vi "BRig_Host_v0,52__noGlobal.vi"() -> ()   [LabVIEW 2014]
uses:
  <vilib>/WebDAVClient/Advanced/SessionHandle.ctl
  BRig_Host__global__stopHost.vi
  <vilib>/Utility/file.llb/Write To Spreadsheet File (DBL).vi
  <vilib>/WebDAVClient/NI_WebDAV.lvlib
panel:
  out "writeError":bool
  out "error IO":errorcluster
  out "error_loopP_loadSettings":errorcluster caption="error out"
  out "testCmdList":u16[][](array[numeric])
  in  "ClosedLoop":bool
  in  "module":string=" module1 "
  in  "input_updateTrial_subsequent":u16
  in  "input_updateTrial_first":u16
  in  "input_forceUpdate":bool
  in  "ClosedLoop":u16[](array[numeric])
  in  "testNewLaserSettings":bool
  in  "LoadSettings":bool
  in  "DisplayNumber":u16
  out "XY Graph":cluster{u16[], u16[]}[](graph)
  in  "threshold_2":u16=600
  in  "threshold_1":u16=300
  in  "Port (F=A/B, T=C)":bool
  out "I_ExpRun":bool
  out "TCP_connection":bool
  in  "stopHost":bool
  # "Port Switch\nToggle TRUE if debugging"
  # "# Trials Displayed\n( 0 = all )"
  # "Selection\nTime Thresholds"
  # "Exp Run\nIn Progress"
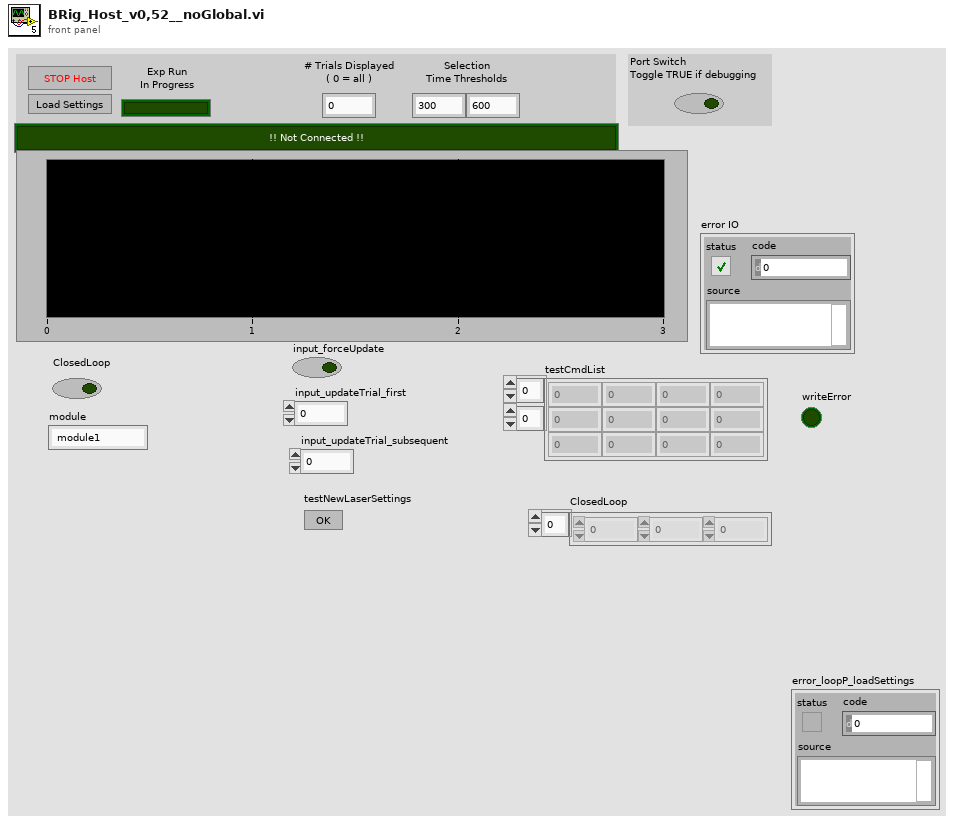
[diagram p1: front panel]
types:
  T1 = typedef "NI_WebDAV.lvlib/SessionHandle.ctl" = refnum<k1>
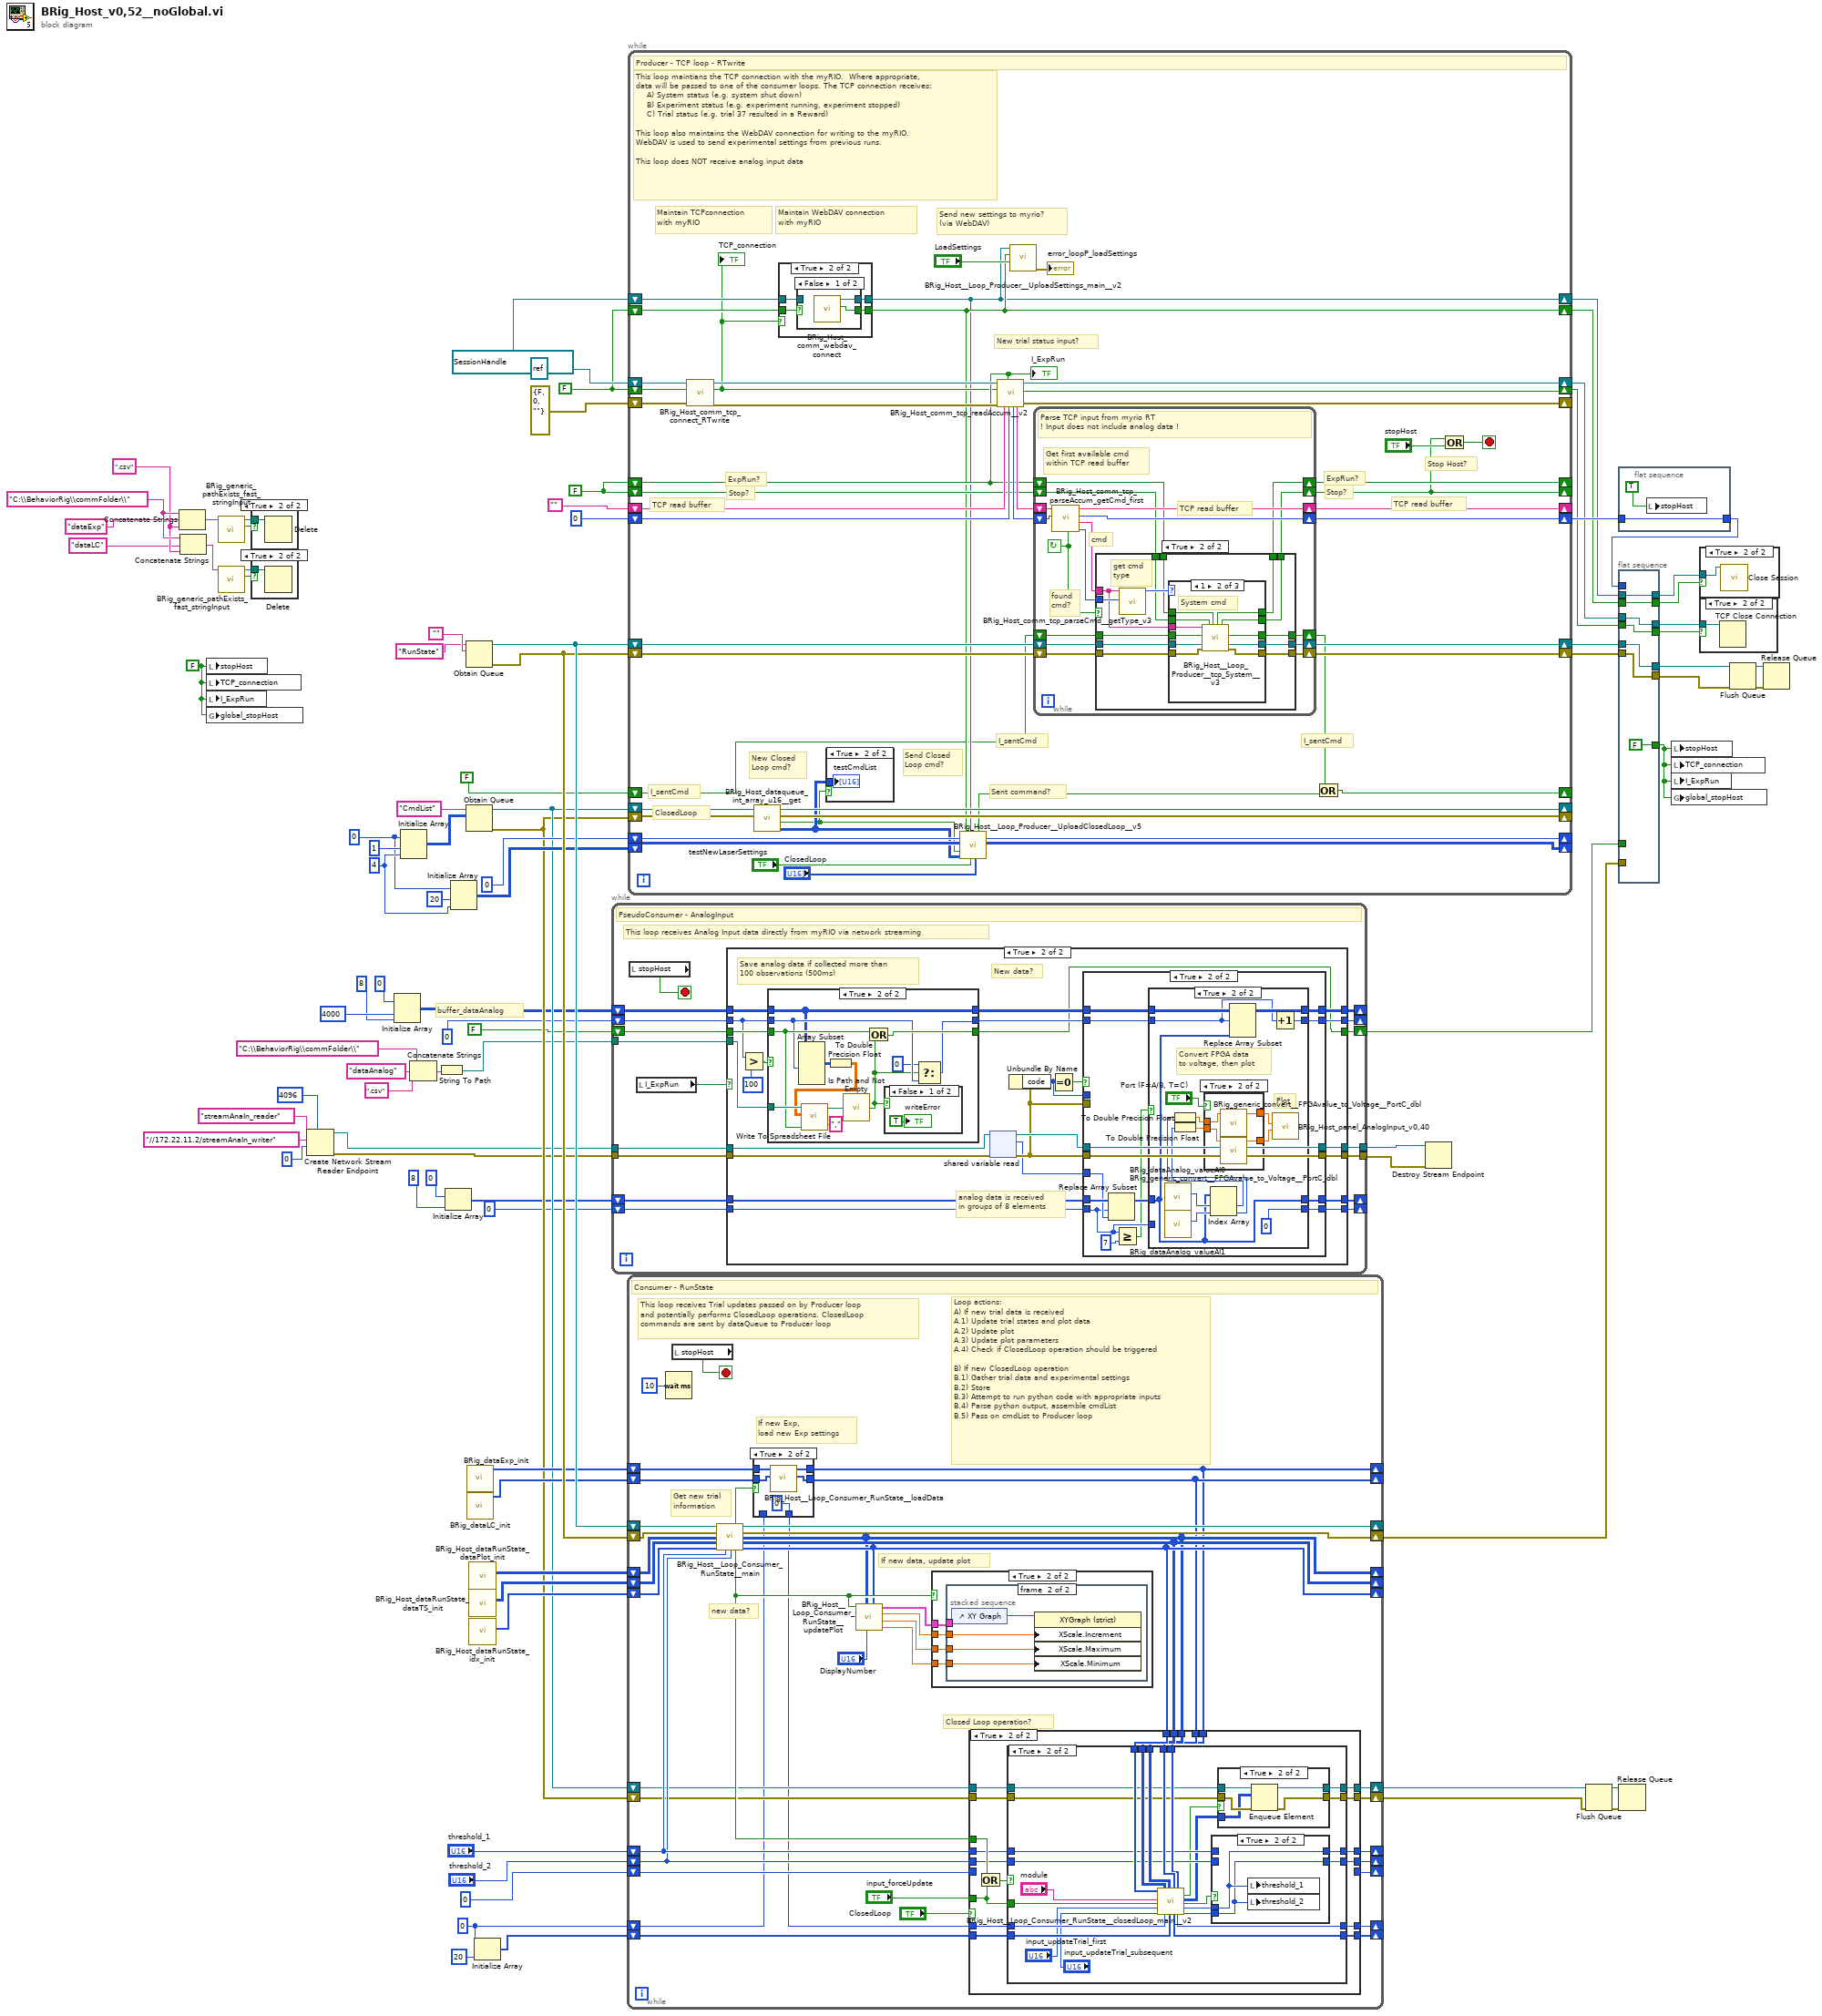
[diagram p0: block diagram]
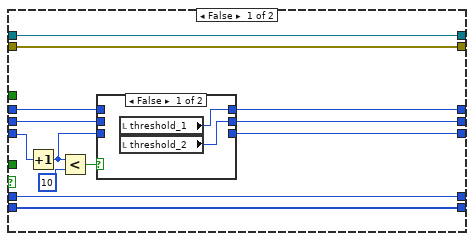
[diagram p6: hidden frame]
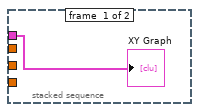
[diagram p13: hidden frame]
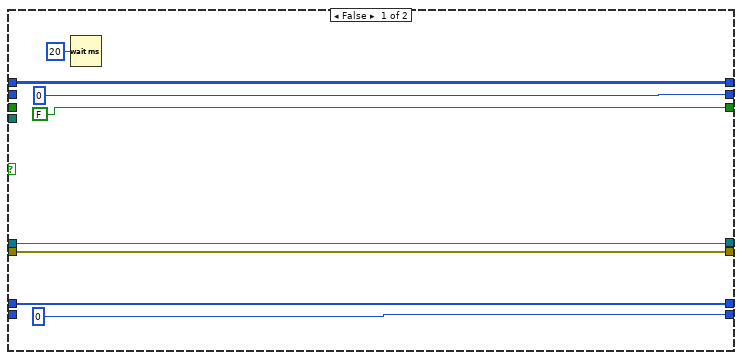
[diagram p14: hidden frame]
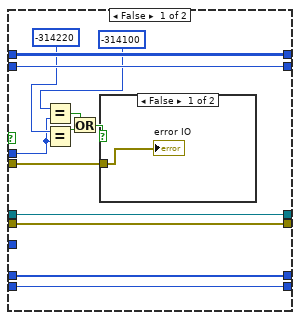
[diagram p15: hidden frame]
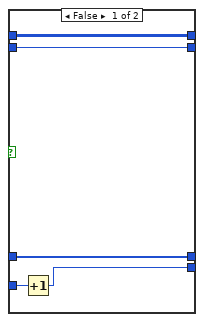
[diagram p17: hidden frame]
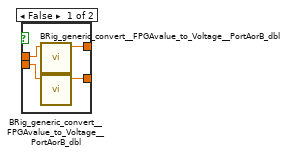
[diagram p18: hidden frame]
diagram:
  w25 = u16 0 ("element")
  w26 = 4 ("dimension size")
  w42 = u16 0
  w54 = ".csv" ("string")
  w55 = "C:\\BehaviorRig\\commFolder\\"
  w67 = T1 refnum items=["Session NI_WebDAV"] ("session handle")
  w85 = FALSE ("stopHost")
  w86 = FALSE
  w68 = FALSE
  # "buffer_dataAnalog"
  n1 = Concatenate Strings(w55, "dataExp" ("string"), w54) -> (w49:string)
  n2 = Concatenate Strings(w55, "dataLC" ("string"), w54) -> (w46:string)
  n3 = local write "stopHost"(w85) -> ()
  n4 = local write "TCP_connection"(w85) -> ()
  n5 = local write "I_ExpRun"(w85) -> ()
  n6 = global write "BRig_Host__global__stopHost.vi" "global_stopHost"(w85) -> ()
  n7 = call "BRig_generic_pathExists_fast_stringInput.vi"("input_filePath"=w49) -> ("output_Iexist"=w51:bool, "output_filePath"=w50:path)  [unwired: 8 in, 1 out]
  n8 = call "BRig_generic_pathExists_fast_stringInput.vi"("input_filePath"=w46) -> ("output_Iexist"=w47:bool, "output_filePath"=w48:path)  [unwired: 8 in, 1 out]
  n9 = case shown="True" w51 {
    tunnel: w50 -> [_ w91]
    frame False {
    }
    frame True {
      n10 = Delete(path (use dialog)=w91) -> ()  [unwired: 4 in, 3 out]
    }
  }
  n11 = case shown="True" w47 {
    tunnel: w48 -> [_ w92]
    frame False {
    }
    frame True {
      n12 = Delete(path (use dialog)=w92) -> ()  [unwired: 4 in, 3 out]
    }
  }
  n13 = Create Network Stream Reader Endpoint(7:4096 ("reader buffer size"), 9:u16 0 ("element"), 10:"//172.22.11.2/streamAnaIn_writer" ("writer url"), 11:"streamAnaIn_reader" ("reader name")) -> (0:w9:errorcluster, 3:w10:refnum<k21>)  [unwired: 3 in]
  n14 = Initialize Array(u16 0 ("element"), 4000 ("dimension size"), 8 ("dimension size")) -> (w21:u16[][])
  n15 = Initialize Array(w25, 1 ("dimension size"), w26) -> (w37:u16[][])
  n16 = Concatenate Strings("C:\\BehaviorRig\\commFolder\\" ("string"), "dataAnalog" ("input_filename"), ".csv" ("string")) -> (w18:string)
  n17 = String To Path(string=w18) -> (path=w15:path)
  n18 = Initialize Array(u16 0 ("element"), 8 ("dimension size")) -> (w2:u16[])
  n19 = Initialize Array(w25, 20 ("dimension size"), w26) -> (w56:u16[][])
  n20 = Obtain Queue(name (unnamed)="RunState", element data type="") -> (queue out=w77:refnum<queue>, error out=w76:errorcluster)  [unwired: 3 in, 1 out]
  n21 = Obtain Queue(name (unnamed)="CmdList", element data type=w37) -> (queue out=w36:refnum<queue>, error out=w35:errorcluster)  [unwired: 3 in, 1 out]
  n22 = call "BRig_dataExp_init.vi"() -> ("output_dataExp"=w45:u16[])  [unwired: 11 in]
  n23 = call "BRig_dataLC_init.vi"() -> ("output_dataLC"=w44:u16[])  [unwired: 11 in]
  n24 = call "BRig_Host_dataRunState_dataPlot_init.vi"() -> ("output_dataPlot"=w73:u16[][])  [unwired: 11 in]
  n25 = call "BRig_Host_dataRunState_dataTS_init.vi"() -> ("output_dataTS"=w72:u16[][])  [unwired: 11 in]
  n26 = call "BRig_Host_dataRunState_idx_init.vi"() -> ("output_idx"=w71:i32[])  [unwired: 11 in]
  n27 = Initialize Array(w42, 20 ("dimension size")) -> (w40:u16[])
  n28 = while {
    shift-right: [w107] -> _
    shift-left: w21 -> [w109]
    shift-right: [w106] -> _
    shift-left: 0 -> [w108]
    tunnel: w15 -> [w105]
    shift-right: [w103] -> w13
    shift-left: FALSE -> [w104]
    tunnel: w10 -> [w101]
    tunnel: w9 -> [w100]
    tunnel: [w99] -> w7
    tunnel: [w98] -> w6
    shift-right: [w95] -> _
    shift-left: w2 -> [w97]
    shift-right: [w94] -> _
    shift-left: 0 ("element") -> [w96]
    stop <- w93 stop-if-true
    # "This loop receives Analog Input data directly from myRIO via network streaming"
    # "PseudoConsumer - AnalogInput"
    n29 = local read "stopHost"() -> (w93:bool)
    n30 = local read "I_ExpRun"() -> (w102:bool)
    n31 = case shown="True" w102 {
      tunnel: w109 -> [w116 w140]
      tunnel: w108 -> [_ w126]
      tunnel: [w116 w135] -> w107
      tunnel: [0 w133] -> w106
      tunnel: w105 -> [_ w138]
      tunnel: w104 -> [_ w139]
      tunnel: [FALSE w123] -> w103
      tunnel: w101 -> [w113 w132]
      tunnel: w100 -> [w112 w131]
      tunnel: [w113 w129] -> w99
      tunnel: [w112 w127] -> w98
      tunnel: w97 -> [w111 w121]
      tunnel: w96 -> [_ w120]
      tunnel: [w111 w119] -> w95
      tunnel: [0 ("element") w118] -> w94
      frame False {
        n32 = Wait (ms)(milliseconds to wait=u32 20) -> ()  [unwired: 1 out]
      }
      frame True {
        # "analog data is received\nin groups of 8 elements"
        # "New data?"
        # "Save analog data if collected more than\n100 observations (500ms)"
        n33 = Greater?(x=w126, y=100) -> (0:w141:bool)
        n34 = case shown="True" w141 {
          tunnel: w140 -> [w200 w203]
          tunnel: [w200 w203] -> w136
          tunnel: w126 -> [w199 w205]
          tunnel: w139 -> [w198 w207]
          tunnel: [w199 w204] -> w134
          tunnel: [w198 w206] -> w123
          tunnel: w138 -> [_ w212]
          frame False {
          }
          frame True {
            n35 = Array Subset(array=w203, length (row)=w205) -> (w211:u16[][])  [unwired: 3 in]
            n36 = To Double Precision Float(number=w211) -> (double precision float=w210:dbl[][])
            n37 = call-poly <vilib>:"Write To Spreadsheet File.vi"("delimiter (\\t)"="," ("delimiter (\\t)"), "append to file? (new file:F)"=w207, "2D data"=w210, "file path (dialog if empty)"=w212) -> ("new file path (Not A Path if cancelled)"=w208:path)  [unwired: 4 in]
            n38 = call <vilib>:"Is Path and Not Empty.vi"("path"=w208) -> ("Is Path and Not Empty?"=w201:bool)  [unwired: 4 in]
            n39 = Or(x=w207, y=w201) -> (x .or. y?=w206:bool)
            n40 = case shown="False" w201 {
              frame False {
                "writeError" <- TRUE ("writeError")
              }
              frame True {
              }
            }
            n41 = Select(t=0, s=w201, f=w205) -> (s? t:f=w204:i32)
          }
        }
        n42 = shared-variable-read(w132, w131) -> (w130:refnum<k21>, w128:errorcluster, w122:u16)  [unwired: 1 in, 1 out]
        n43 = Unbundle By Name(w128) -> ("code"=w124:i32)
        n44 = Equal To 0?(x=w124) -> (x = 0?=w137:bool)
        n45 = case shown="True" w137 {
          tunnel: w136 -> [w154 w169]
          tunnel: [w154 w168] -> w135
          tunnel: w134 -> [w153 w167]
          tunnel: [w153 w166] -> w133
          tunnel: w128 -> [w151 _]
          tunnel: w130 -> [w150 w165]
          tunnel: [w150 w165] -> w129
          tunnel: w128 -> [w149 w164]
          tunnel: [w149 w164] -> w127
          tunnel: w124 -> [w148 _]
          tunnel: w122 -> [_ w162]
          tunnel: w121 -> [w143 w163]
          tunnel: w120 -> [w142 w160]
          tunnel: [w143 w157] -> w119
          tunnel: [w142 w159] -> w118
          frame False {
            n46 = Equal?(x=-314100, y=w148) -> (x = y?=w146:bool)
            n47 = Equal?(x=-314220, y=w148) -> (x = y?=w145:bool)
            n48 = Or(x=w146, y=w145) -> (x .or. y?=w144:bool)
            n49 = case shown="False" w144 {
              tunnel: w151 -> [w155 _]
              frame False {
                "error IO" <- w155
              }
              frame True {
              }
            }
          }
          frame True {
            n50 = Replace Array Subset(array=w163, new element=w162, index=w160) -> (w158:u16[])
            n51 = Greater Or Equal?(x=w160, y=7) -> (x >= y?=w156:bool)
            n52 = case shown="True" w156 {
              tunnel: w169 -> [w174 w189]
              tunnel: [w174 w188] -> w168
              tunnel: w167 -> [w173 w187]
              tunnel: [w173 w186] -> w166
              tunnel: w160 -> [w172 _]
              tunnel: [w171 0 ("y")] -> w159
              tunnel: w158 -> [w170 w177]
              tunnel: [w170 w177] -> w157
              frame False {
                n53 = Increment(x=w172) -> (x+1=w171:i32)
              }
              frame True {
                # "Convert FPGA data\nto voltage, then plot"
                # "Plot"
                n54 = call "BRig_dataAnalog_valueAI0.vi"() -> ("output_valueAI0"=w179:i32)  [unwired: 11 in]
                n55 = call "BRig_dataAnalog_valueAI1.vi"() -> ("output_valueAI1"=w180:i32)  [unwired: 11 in]
                n56 = Index Array(array=w177, index #1=w179, index #2=w180) -> (element #1=w176:u16, element #2=w175:u16)
                n57 = To Double Precision Float(number=w176) -> (double precision float=w181:dbl)
                n58 = To Double Precision Float(number=w175) -> (double precision float=w182:dbl)
                n59 = case shown="True" "Port (F=A/B, T=C)" {
                  tunnel: w181 -> [w191 w197]
                  tunnel: w182 -> [w190 w196]
                  tunnel: [w193 w195] -> w184
                  tunnel: [w192 w194] -> w183
                  frame False {
                    n60 = call "BRig_generic_convert__FPGAvalue_to_Voltage__PortAorB_dbl.vi"("input_FPGAvalue_PortAorB"=w191) -> ("output_voltage"=w193:dbl)  [unwired: 10 in]
                    n61 = call "BRig_generic_convert__FPGAvalue_to_Voltage__PortAorB_dbl.vi"("input_FPGAvalue_PortAorB"=w190) -> ("output_voltage"=w192:dbl)  [unwired: 10 in]
                  }
                  frame True {
                    n62 = call "BRig_generic_convert__FPGAvalue_to_Voltage__PortC_dbl.vi"("input_FPGAvalue_PortC"=w197) -> ("output_voltage"=w195:dbl)  [unwired: 10 in]
                    n63 = call "BRig_generic_convert__FPGAvalue_to_Voltage__PortC_dbl.vi"("input_FPGAvalue_PortC"=w196) -> ("output_voltage"=w194:dbl)  [unwired: 10 in]
                  }
                }
                n64 = Replace Array Subset(array=w189, new element=w177, index (row)=w187) -> (w188:u16[][])  [unwired: 1 in]
                n65 = Increment(x=w187) -> (x+1=w186:i32)
                n66 = call "BRig_Host_panel_AnalogInput_v0,40.vi"("graph_ai1"=w183, "graph_ai0"=w184) -> ()  [unwired: 10 in]
              }
            }
          }
        }
      }
    }
  }
  n67 = while {
    shift-right: [w246] -> _
    shift-left: w77 -> [w247]
    shift-right: [w244] -> w30
    shift-left: w76 -> [w245]
    shift-right: [w227] -> _
    shift-left: w73 -> [w243]
    shift-right: [w228] -> _
    shift-left: w72 -> [w242]
    shift-right: [w229] -> _
    shift-left: w71 -> [w241]
    shift-right: [w237] -> _
    shift-left: "threshold_1" -> [w236]
    shift-right: [w235] -> _
    shift-left: "threshold_2" -> [w234]
    shift-right: [w225] -> _
    shift-left: w45 -> [w239]
    shift-right: [w226] -> _
    shift-left: w44 -> [w238]
    shift-right: [w219] -> _
    shift-left: w42 -> [w217]
    shift-right: [w231] -> _
    shift-left: u8 0 -> [w232]
    shift-right: [w218] -> _
    shift-left: w40 -> [w215]
    shift-right: [w222] -> w32
    shift-left: w36 -> [w224]
    shift-right: [w221] -> w31
    shift-left: w35 -> [w223]
    stop <- w214 stop-if-true
    # "Closed Loop operation?"
    # "Loop actions:\nA) If new trial data is received\nA.1) Update trial states and plot data\nA.2) Update plot\nA.3) Update plot parameters\nA.4) Check if ClosedLoop operation should be triggered\n\nB) If new ClosedLoop operation\nB.1) Gather trial data and experimental settings\nB.2) Store\nB.3) Attempt to run python code with appropriate inputs\nB.4) Parse python output, assemble cmdList\nB.5) Pass on cmdList to Producer loop"
    # "This loop receives Trial updates passed on by Producer loop\nand potentially performs ClosedLoop operations. ClosedLoop\ncommands are sent by dataQueue to Producer loop"
    # "If new data, update plot"
    # "If new Exp,\nload new Exp settings"
    # "new data?"
    # "Get new trial\ninformation"
    # "Consumer - RunState"
    n68 = Wait (ms)(milliseconds to wait=u32 10) -> ()  [unwired: 1 out]
    n69 = local read "stopHost"() -> (w214:bool)
    n70 = call "BRig_Host__Loop_Consumer_RunState__main.vi"("input_hDataQueue"=w247, "input_errorDataQueue"=w245, "input_dataPlot"=w243, "input_dataTS"=w242, "input_idx"=w241, "threshold_1"=w236, "threshold_2"=w234) -> ("output_ExpStart"=w240:bool, "output_hDataQueue"=w246:refnum<queue>, "output_errorDataQueue"=w244:errorcluster, "output_dataPlot"=w227:u16[][], "output_dataTS"=w228:u16[][], "output_updatePlot"=w230:bool, "output_idx"=w229:i32[])  [unwired: 2 in]
    n71 = case shown="True" w240 {
      tunnel: w239 -> [w337 w339]
      tunnel: [w337 w342] -> w225
      tunnel: w238 -> [w336 w340]
      tunnel: [w336 w341] -> w226
      tunnel: w217 -> [w335 _]
      tunnel: [w335 u16 0] -> w216
      frame False {
      }
      frame True {
        n72 = call "BRig_Host__Loop_Consumer_RunState__loadData.vi"("input_dataLC"=w340, "input_dataExp"=w339) -> ("output_dataLC"=w341:u16[], "output_dataExp"=w342:u16[])  [unwired: 8 in]
      }
    }
    n73 = call "BRig_Host__Loop_Consumer_RunState__updatePlot.vi"("input_idx"=w229, "input_DisplayNumber"="DisplayNumber", "input_dataPlot"=w227, "input_updatePlot"=w230) -> ("output_X_min"=w250:dbl, "output_X_max"=w249:dbl, "output_X_inc"=w248:dbl, "XY Graph"=w251:cluster{u16[], u16[]}[])  [unwired: 4 in]
    n74 = case shown="True" w230 {
      tunnel: w251 -> [_ w346]
      tunnel: w250 -> [_ w345]
      tunnel: w249 -> [_ w344]
      tunnel: w248 -> [_ w343]
      frame False {
      }
      frame True {
        n75 = stacked-sequence {
          tunnel: w346 -> [w347 _]
          tunnel: w345 -> [_ w350]
          tunnel: w344 -> [_ w349]
          tunnel: w343 -> [_ w348]
          frame #0 {
            "XY Graph" <- w347
          }
          frame #1 {
            n76 = control-ref of="XY Graph"() -> (w351:refnum<vi>)
            n77 = property class="XYGraph (strict)"(reference=w351, "XScale.Increment"=w348, "XScale.Maximum"=w349, "XScale.Minimum"=w350) -> ()  [unwired: 1 in, 2 out]
          }
        }
      }
    }
    n78 = case shown="True" "ClosedLoop" {
      tunnel: [w261 w284] -> w237
      tunnel: w236 -> [w262 w285]
      tunnel: [w260 w282] -> w235
      tunnel: w234 -> [w263 w283]
      tunnel: w232 -> [w266 _]
      tunnel: [w259 _] -> w231
      tunnel: w216 -> [w257 w289]
      tunnel: [w257 w287] -> w219
      tunnel: w215 -> [w256 w288]
      tunnel: [w256 w286] -> w218
      tunnel: w230 -> [_ w291]
      tunnel: w229 -> [_ w281]
      tunnel: w228 -> [_ w280]
      tunnel: w227 -> [_ w279]
      tunnel: w226 -> [_ w278]
      tunnel: w225 -> [_ w277]
      tunnel: w224 -> [w255 w276]
      tunnel: w223 -> [w254 w275]
      tunnel: [w255 w274] -> w222
      tunnel: [w254 w273] -> w221
      tunnel: "input_forceUpdate" -> [_ w272]
      frame False {
        n79 = Increment(x=w266) -> (x+1=w258:u8)
        n80 = Less?(x=w258, y=u8 10) -> (x < y?=w264:bool)
        n81 = case shown="False" w264 {
          tunnel: w263 -> [_ w270]
          tunnel: w262 -> [_ w271]
          tunnel: [w268 w271] -> w261
          tunnel: [w267 w270] -> w260
          tunnel: [_ w269] -> w259
          tunnel: w258 -> [_ w269]
          frame False {
            n82 = local read "threshold_1"() -> (w268:u16)
            n83 = local read "threshold_2"() -> (w267:u16)
          }
          frame True {
          }
        }
      }
      frame True {
        n84 = Or(x=w291, y=w272) -> (x .or. y?=w290:bool)
        n85 = case shown="True" w290 {
          tunnel: w272 -> [_ w320]
          tunnel: w289 -> [w297 w323]
          tunnel: w288 -> [w296 w322]
          tunnel: [w297 w316] -> w287
          tunnel: [w296 w317] -> w286
          tunnel: w285 -> [w295 w310]
          tunnel: [w295 w306] -> w284
          tunnel: w283 -> [w294 w309]
          tunnel: [w294 w305] -> w282
          tunnel: w281 -> [_ w315]
          tunnel: w280 -> [_ w314]
          tunnel: w279 -> [_ w313]
          tunnel: w278 -> [_ w312]
          tunnel: w277 -> [_ w311]
          tunnel: w276 -> [w293 w303]
          tunnel: w275 -> [w292 w301]
          tunnel: [w293 w302] -> w274
          tunnel: [w292 w300] -> w273
          frame False {
          }
          frame True {
            n86 = call "BRig_Host__Loop_Consumer_RunState__closedLoop_main__v2.vi"("input_idx"=w315, "input_module"="module", "input_forceUpdate"=w320, "input_updateTrial_first"="input_updateTrial_first", "input_updateTrial_subsequent"="input_updateTrial_subsequent", "input_dataTS"=w314, "input_updateID"=w323, "input_dataPlot"=w313, "input_trialList"=w322, "input_dataLC"=w312, "input_dataExp"=w311) -> ("output_trialList"=w317:u16[], "output_updateID"=w316:u16, 15:"output_cmdList"=w298:bool, 16:"output_cmdList"=w299:u16[][], "output_thres"=w304:bool, "output_thres1"=w308:u16, "output_thres2"=w307:u16)  [unwired: 2 in]
            n87 = case shown="True" w304 {
              tunnel: w310 -> [w332 _]
              tunnel: w309 -> [w331 _]
              tunnel: w308 -> [_ w334]
              tunnel: w307 -> [_ w333]
              tunnel: [w332 w334] -> w306
              tunnel: [w331 w333] -> w305
              frame False {
              }
              frame True {
                n88 = local write "threshold_1"(w334) -> ()
                n89 = local write "threshold_2"(w333) -> ()
              }
            }
            n90 = case shown="True" w298 {
              tunnel: w303 -> [w325 w330]
              tunnel: [w325 w327] -> w302
              tunnel: w301 -> [w324 w329]
              tunnel: [w324 w326] -> w300
              tunnel: w299 -> [_ w328]
              frame False {
              }
              frame True {
                n91 = Enqueue Element(queue=w330, element=w328, error in (no error)=w329) -> (queue out=w327:refnum<queue>, error out=w326:errorcluster)  [unwired: 1 in, 1 out]
              }
            }
          }
        }
      }
    }
  }
  n92 = while {
    shift-right: [w378] -> w61
    shift-left: w68 -> [w398]
    shift-right: [w393] -> w62
    shift-left: refnum<k5> refnum ("output_hTCP") -> [w397]
    shift-right: [w392] -> _
    shift-left: errorcluster {"status"=FALSE, "code"=0, "source"=""} ("output_error") -> [w396]
    shift-right: [w387] -> _
    shift-left: "" ("input_strAccum") -> [w391]
    shift-right: [w386] -> w75
    shift-left: 0 ("input_count") -> [w390]
    shift-right: [w385] -> _
    shift-left: w86 -> [w363]
    shift-right: [w361] -> _
    shift-left: w86 -> [w383]
    shift-right: [w380] -> w81
    shift-left: w77 -> [w382]
    shift-right: [w379] -> w80
    shift-left: w76 -> [w381]
    shift-right: [w358] -> w66
    shift-left: w68 -> [w377]
    shift-right: [w357] -> w65
    shift-left: w67 -> [w376]
    shift-right: [w368] -> _
    shift-left: w56 -> [w369]
    shift-right: [w352] -> _
    shift-left: 0 -> [w370]
    shift-right: [w372] -> _
    shift-left: w36 -> [w374]
    shift-right: [w371] -> _
    shift-left: w35 -> [w373]
    shift-right: [w353] -> _
    shift-left: FALSE -> [w356]
    stop <- w360 stop-if-true
    # "ClosedLoop"
    # "TCP read buffer"
    # "TCP read buffer"
    # "I_sentCmd"
    # "Sent command?"
    # "I_sentCmd"
    # "I_sentCmd"
    # "Stop Host?"
    # "Send Closed\nLoop cmd?"
    # "New Closed\nLoop cmd?"
    # "New trial status input?"
    # "ExpRun?"
    # "Stop?"
    # "This loop maintians the TCP connection with the myRIO.  Where appropriate,\ndata will be passed to one of the consumer loops. The TCP connection receives:\n    A) System status (e.g. system shut down)\n    B) Experiment status (e.g. experiment running, experiment stopped)\n    C) Trial status (e.g. trial 37 resulted in a Reward)\n\nThis loop also maintains the WebDAV connection for writing to the myRIO.\nWebDAV is used to send experimental settings from previous runs.\n\nThis loop does NOT receive analog input data"
    # "Send new settings to myrio?\n(via WebDAV)"
    # "ExpRun?"
    # "Stop?"
    # "Maintain TCPconnection\nwith myRIO"
    # "Maintain WebDAV connection\nwith myRIO"
    # "Producer - TCP loop - RTwrite"
    n93 = call "BRig_Host_comm_tcp_connect_RTwrite.vi"("input_error"=w396, "input_connected"=w398, "input_hTCP"=w397) -> ("output_error"=w394:errorcluster, "output_connected"=w362:bool, "output_hTCP"=w395:refnum<k5>)  [unwired: 5 in, 1 out]
    "TCP_connection" <- w362
    n94 = call "BRig_Host_dataqueue_int_array_u16__get.vi"("input_erroDataQueue"=w373, "input_hDataQueue"=w374) -> (0:"output_data"=w365:u16[][], 1:"output_data"=w364:bool, "output_errorDataQueue"=w371:errorcluster, "output_hDataQueue"=w372:refnum<queue>)  [unwired: 6 in]
    n95 = case shown="True" w362 {
      tunnel: w377 -> [w403 w411]
      tunnel: [w402 w410] -> w358
      tunnel: w376 -> [w401 w409]
      tunnel: [w400 w408] -> w357
      frame False {
        n96 = case shown="True" w403 {
          selector: w403 -> [w405 _]
          tunnel: [w405 FALSE] -> w402
          tunnel: w401 -> [w404 w406]
          tunnel: [w404 _] -> w400
          frame False {
          }
          frame True {
            n97 = call <vilib>:"Close Session.vi"("session handle"=w406) -> ()  [unwired: 14 in, 1 out]
          }
        }
      }
      frame True {
        n98 = case shown="False" w411 {
          selector: w411 -> [_ w415]
          tunnel: [w412 w415] -> w410
          tunnel: w409 -> [_ w414]
          tunnel: [w413 w414] -> w408
          frame False {
            n99 = call "BRig_Host_comm_webdav_connect.vi"() -> ("output_Iconnected"=w412:bool, "output_hSession"=w413:T1)  [unwired: 9 in, 1 out]
          }
          frame True {
          }
        }
      }
    }
    n100 = case shown="True" w364 {
      tunnel: w365 -> [_ w399]
      frame False {
      }
      frame True {
        "testCmdList" <- w399
      }
    }
    n101 = call "BRig_Host__Loop_Producer__UploadClosedLoop__v5.vi"("input_arrayBuffer_length"=w370, "input_arrayBuffer"=w369, 4:"input_cmdList"=w364, 5:"input_cmdList"=w365, "input_webdav_status"=w358, "session handle"=w357, "testNewLaserSettings"="testNewLaserSettings", "input_array_LaserSettings"="ClosedLoop") -> ("Sent"=w354:bool, "output_arrayBuffer_length"=w352:i32, "output_arrayBuffer"=w368:u16[][])  [unwired: 9 in]
    n102 = call "BRig_Host_comm_tcp_readAccum__v2.vi"("input_handle_TCP"=w395, "input_connected"=w362, "input_error"=w394, "input_strAccum"=w391, "input_I_ExpRun"=w363, "input_count"=w390) -> ("output_count"=w388:i32, "output_strAccum"=w389:string, "output_handle_TCP"=w393:refnum<k5>, "output_connected"=w378:bool, "output_error"=w392:errorcluster)  [unwired: 9 in]
    n103 = call "BRig_Host__Loop_Producer__UploadSettings_main__v2.vi"("input_LoadSettings"="LoadSettings", "input_webdav_status"=w358, "session handle"=w357) -> ("error out"=→"error_loopP_loadSettings":errorcluster)  [unwired: 8 in]
    n104 = while {
      shift-right: [w429] -> w387
      shift-left: w389 -> [w432]
      shift-right: [w428] -> w386
      shift-left: w388 -> [w431]
      shift-right: [w424] -> w385
      shift-left: w363 -> [w425]
      shift-right: [w422] -> w361
      shift-left: w383 -> [w423]
      shift-right: [w418] -> w380
      shift-left: w382 -> [w421]
      shift-right: [w419] -> w379
      shift-left: w381 -> [w420]
      shift-right: [w416] -> w355
      shift-left: w356 -> [w417]
      stop <- w430 continue-if-true
      # "found\ncmd?"
      # "TCP read buffer"
      # "cmd"
      # "Get first available cmd\nwithin TCP read buffer"
      # "Parse TCP input from myrio RT\n! Input does not include analog data !"
      n105 = call "BRig_Host_comm_tcp_parseAccum_getCmd_first.vi"("input_count"=w431, "input_strAccum"=w432) -> ("output_countCmd"=w426:i32, "output_strCmd"=w427:string, "output_count"=w428:i32, "output_strAccum"=w429:string, "output_I_cmd"=w430:bool)  [unwired: 5 in]
      n106 = case shown="True" w430 {
        tunnel: w427 -> [_ w448]
        tunnel: w426 -> [_ w450]
        tunnel: w425 -> [w437 w443]
        tunnel: [w437 w441] -> w424
        tunnel: w423 -> [w436 w442]
        tunnel: [w436 w440] -> w422
        tunnel: w421 -> [w435 w447]
        tunnel: w420 -> [w434 w446]
        tunnel: [w434 w445] -> w419
        tunnel: [w435 w444] -> w418
        tunnel: w417 -> [w433 w439]
        tunnel: [w433 w438] -> w416
        frame False {
        }
        frame True {
          # "get cmd\ntype"
          n107 = call "BRig_Host_comm_tcp_parseCmd__getType_v3.vi"("input_strCmd"=w448, "input_countCmd"=w450) -> ("output_strType"=w449:u8)  [unwired: 17 in]
          n108 = case shown="1" w449 {
            tunnel: w448 -> [_ w462 w474]
            tunnel: w447 -> [w455 w465 w473]
            tunnel: w446 -> [w454 w466 w472]
            tunnel: [w454 w464 w471] -> w445
            tunnel: [w455 w463 w470] -> w444
            tunnel: w443 -> [w453 w461 w469]
            tunnel: w442 -> [w452 w460 w468]
            tunnel: [w453 w459 w469] -> w441
            tunnel: [w452 w458 w468] -> w440
            tunnel: w439 -> [w451 w457 w467]
            tunnel: [w451 w456 w467] -> w438
            frame 0, Default {
              # "unknown cmd"
            }
            frame 1 {
              # "System cmd"
              n109 = call "BRig_Host__Loop_Producer__tcp_System__v3.vi"("input_strCmd"=w462, "input_I_SentCmd"=w457, "input_hDataQueue"=w465, "input_error_dataqueue"=w466, "input_I_Stop"=w460, "input_I_ExpRun"=w461) -> ("output_I_ExpRun"=w459:bool, "output_I_Stop"=w458:bool, "output_I_sentCmd"=w456:bool, "output_hDataQueue"=w463:refnum<queue>, "output_error"=w464:errorcluster)  [unwired: 9 in]
            }
            frame 2 {
              # "Send to\nconsumer loop"
              # "Trial state cmd"
              n110 = Enqueue Element(queue=w473, element=w474, error in (no error)=w472) -> (queue out=w470:refnum<queue>, error out=w471:errorcluster)  [unwired: 1 in, 1 out]
            }
          }
        }
      }
    }
    n111 = Or(x=w355, y=w354) -> (x .or. y?=w353:bool)
    n112 = Or(x=w361, y="stopHost") -> (x .or. y?=w360:bool)
    "I_ExpRun" <- w363
  }
  n113 = Destroy Stream Endpoint(8:w6, 11:w7) -> ()  [unwired: 1 out]
  n114 = Flush Queue(queue=w32, error in (no error)=w31) -> (queue out=w34:refnum<queue>, error out=w33:errorcluster)  [unwired: 1 out]
  n115 = flat-sequence {
    tunnel: w75 -> [w476]
    tunnel: [w476] -> w74
    frame #0 {
      n116 = local write "stopHost"(TRUE ("global_stopHost")) -> ()
    }
  }
  n117 = flat-sequence {
    tunnel: [FALSE] -> w84
    tunnel: w81 -> [w482]
    tunnel: w80 -> [w481]
    tunnel: [w482] -> w79
    tunnel: [w481] -> w78
    tunnel: w74 -> [_]
    tunnel: w66 -> [w479]
    tunnel: w65 -> [w480]
    tunnel: [w480] -> w63
    tunnel: [w479] -> w64
    tunnel: w62 -> [w477]
    tunnel: w61 -> [w478]
    tunnel: [w478] -> w60
    tunnel: [w477] -> w59
    tunnel: w30 -> [_]
    tunnel: w13 -> [_]
    frame #0 {
    }
  }
  n118 = Release Queue(queue=w34, error in (no error)=w33) -> ()  [unwired: 1 in, 3 out]
  n119 = local write "stopHost"(w84) -> ()
  n120 = local write "TCP_connection"(w84) -> ()
  n121 = local write "I_ExpRun"(w84) -> ()
  n122 = global write "BRig_Host__global__stopHost.vi" "global_stopHost"(w84) -> ()
  n123 = case shown="True" w64 {
    tunnel: w63 -> [_ w484]
    frame False {
    }
    frame True {
      n124 = call <vilib>:"Close Session.vi"("session handle"=w484) -> ()  [unwired: 14 in, 1 out]
    }
  }
  n125 = case shown="True" w60 {
    tunnel: w59 -> [_ w485]
    frame False {
    }
    frame True {
      n126 = TCP Close Connection(connection ID=w485) -> ()  [unwired: 2 in, 2 out]
    }
  }
  n127 = Flush Queue(queue=w79, error in (no error)=w78) -> (queue out=w29:refnum<queue>, error out=w28:errorcluster)  [unwired: 1 out]
  n128 = Release Queue(queue=w29, error in (no error)=w28) -> ()  [unwired: 1 in, 3 out]
